vi "Normalise.vi"(3 "min":dbl format="%#_13g", 4 "value":dbl format="%#_13g", 5 "max":dbl format="%#_13g") -> (0 "min":bool, 1 "normalised":dbl, 2 "max":bool)   [LabVIEW 2016]
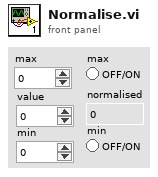
[diagram p1: front panel]
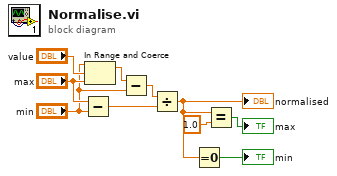
[diagram p0: block diagram]
diagram:
  n1 = Subtract(x="max", y="min") -> (x-y=w6:dbl)
  n2 = In Range and Coerce(upper limit="min", x="value", lower limit="max") -> (coerced(x)=w9:dbl)  [unwired: 1 out]
  n3 = Subtract(x=w9, y="min") -> (x-y=w5:dbl)
  n4 = Divide(x=w5, y=w6) -> (x/y=w3:dbl)
  "normalised" <- w3
  n5 = Equal To 0?(x=w3) -> (x = 0?=→"min":bool)
  n6 = Equal?(x=w3, y=1.0) -> (x = y?=→"max":bool)
